vi "Run (G-Audio).vi"(8 "error in (no error)":errorcluster, 11 "Audio Output Queue":refnum<queue>) -> (0 "error out":errorcluster)   [LabVIEW 2020, in "Audio Output.lvlib"]
doc: "The main audio output loop.\n\n<b>Priority:</b> Time Critical\n<b>Execution System:</b> Instrument I/O"
uses:
  Audio Output.lvlib
  Audio Output Queue Type.ctl
  Audio Output Config.ctl
  Audio Output Info.ctl
  <vilib>/Dataflow_G/G-Audio/Controls/Audio Device Info.ctl
  <vilib>/Dataflow_G/G-Audio/Controls/Audio Device Type.ctl
  <vilib>/Dataflow_G/G-Audio/Controls/Audio Device Native Data Format.ctl
  <vilib>/Dataflow_G/G-Audio/Controls/Audio Device Format.ctl
  State.ctl
  <vilib>/Dataflow_G/G-Audio/Controls/Audio Device Config.ctl
  <vilib>/Dataflow_G/G-Audio/Controls/Audio Device Refnum.ctl
  Packed Libraries/Messaging.lvlibp/Message Cluster.ctl
  0d524fd1-6f2e-443a-bc5a-9f55547fbf75.vi
  df8da7fd-5bea-41c3-a497-f65be9ea8de3.vi
  3674f1a7-3d32-4f10-b3d2-182b6974db2a.vi
  <vilib>/Dataflow_G/G-Audio/Private/Result To Error.vi
  df8da7fd-5bea-41c3-a497-f65be9ea8de3.vi/4dfb5711-8d81-45a3-b3db-a84d40650863.vi
  df8da7fd-5bea-41c3-a497-f65be9ea8de3.vi/c8869513-30c6-44f2-a2d3-73232fe63870.vi
  <vilib>/Dataflow_G/G-Audio/Private/Audio Device Refnum To Value.vi
  3674f1a7-3d32-4f10-b3d2-182b6974db2a.vi/4dfb5711-8d81-45a3-b3db-a84d40650863.vi
  3674f1a7-3d32-4f10-b3d2-182b6974db2a.vi/c8869513-30c6-44f2-a2d3-73232fe63870.vi
  df8da7fd-5bea-41c3-a497-f65be9ea8de3.vi/4dfb5711-8d81-45a3-b3db-a84d40650863.vi/4b7b629c-2e91-4160-9820-a26af8f6e677.vi
  df8da7fd-5bea-41c3-a497-f65be9ea8de3.vi/c8869513-30c6-44f2-a2d3-73232fe63870.vi/4b7b629c-2e91-4160-9820-a26af8f6e677.vi
  3674f1a7-3d32-4f10-b3d2-182b6974db2a.vi/4dfb5711-8d81-45a3-b3db-a84d40650863.vi/4b7b629c-2e91-4160-9820-a26af8f6e677.vi
  3674f1a7-3d32-4f10-b3d2-182b6974db2a.vi/c8869513-30c6-44f2-a2d3-73232fe63870.vi/4b7b629c-2e91-4160-9820-a26af8f6e677.vi
  Packed Libraries/Globals.lvlibp/Constants.vi
  Packed Libraries/Globals.lvlibp/Debug.vi
  <vilib>/Utility/Data Type/Get Numeric Information.vi
  <vilib>/Utility/error.llb/Error Cluster From Error Code.vi
  Packed Libraries/Messaging.lvlibp
  Packed Libraries/Globals.lvlibp
  <vilib>/ptbypt/NI_PtbyPt.lvlib
  <vilib>/Dataflow_G/G-Audio/G-Audio.lvlib
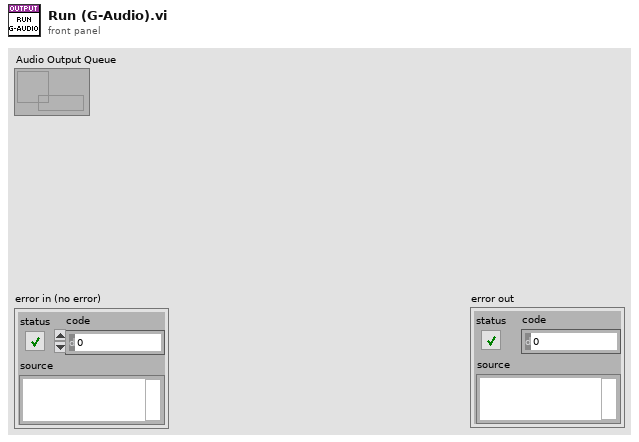
[diagram p1: front panel]
types:
  T1 = typedef "Audio Output.lvlib/Audio Output Config.ctl" = cluster{"Master":T2, "Headphones":T2}
  T2 = typedef "Audio Output.lvlib/Audio Output Info.ctl" = cluster{"Enable":bool, "Device Info":T3}
  T3 = typedef "G-Audio.lvlib/Audio Device Info.ctl" = cluster{"Name":string, "ID":u8[], "Device Type":T4, "Default":bool, "Native Data Formats":T5[]}
  T4 = typedef "G-Audio.lvlib/Audio Device Type.ctl" = enum16{"(None)", "Playback", "Capture", "Duplex", "Loopback"}
  T5 = typedef "G-Audio.lvlib/Audio Device Native Data Format.ctl" = cluster{"Format":T6, "Channels":u32, "Sample Rate (Hz)":u32, "Exclusive Mode":bool}
  T6 = typedef "G-Audio.lvlib/Audio Device Format.ctl" = enum16{"Native", "U8", "I16", "I32", "SGL"}
  T7 = typedef "Audio Output.lvlib/State.ctl" = enum16{"Init", "Configure", "Output", "Error", "Stop", "Idle", "Shutdown"}
  T8 = typedef "G-Audio.lvlib/Audio Device Config.ctl" = cluster{"Sample Rate (Hz)":u32, "Channels":u32, "Format":T6}
  T9 = typedef "G-Audio.lvlib/Audio Device Refnum.ctl" = refnum<file>
  T10 = typedef "Messaging.lvlibp/Message Cluster.ctl" = cluster{"Event":string, "Source":string, "Target":string, "Data":variant}
  T11 = typedef "Messaging.lvlib/Message Cluster.ctl" = cluster{"Event":string, "Source":string, "Target":string, "Data":variant}
  T12 = typedef "Audio Output.lvlib/Audio Output Queue Type.ctl" = cluster{"Master":waveform(i16)[], "Headphones":waveform(i16)[], "Start Time":dbl}
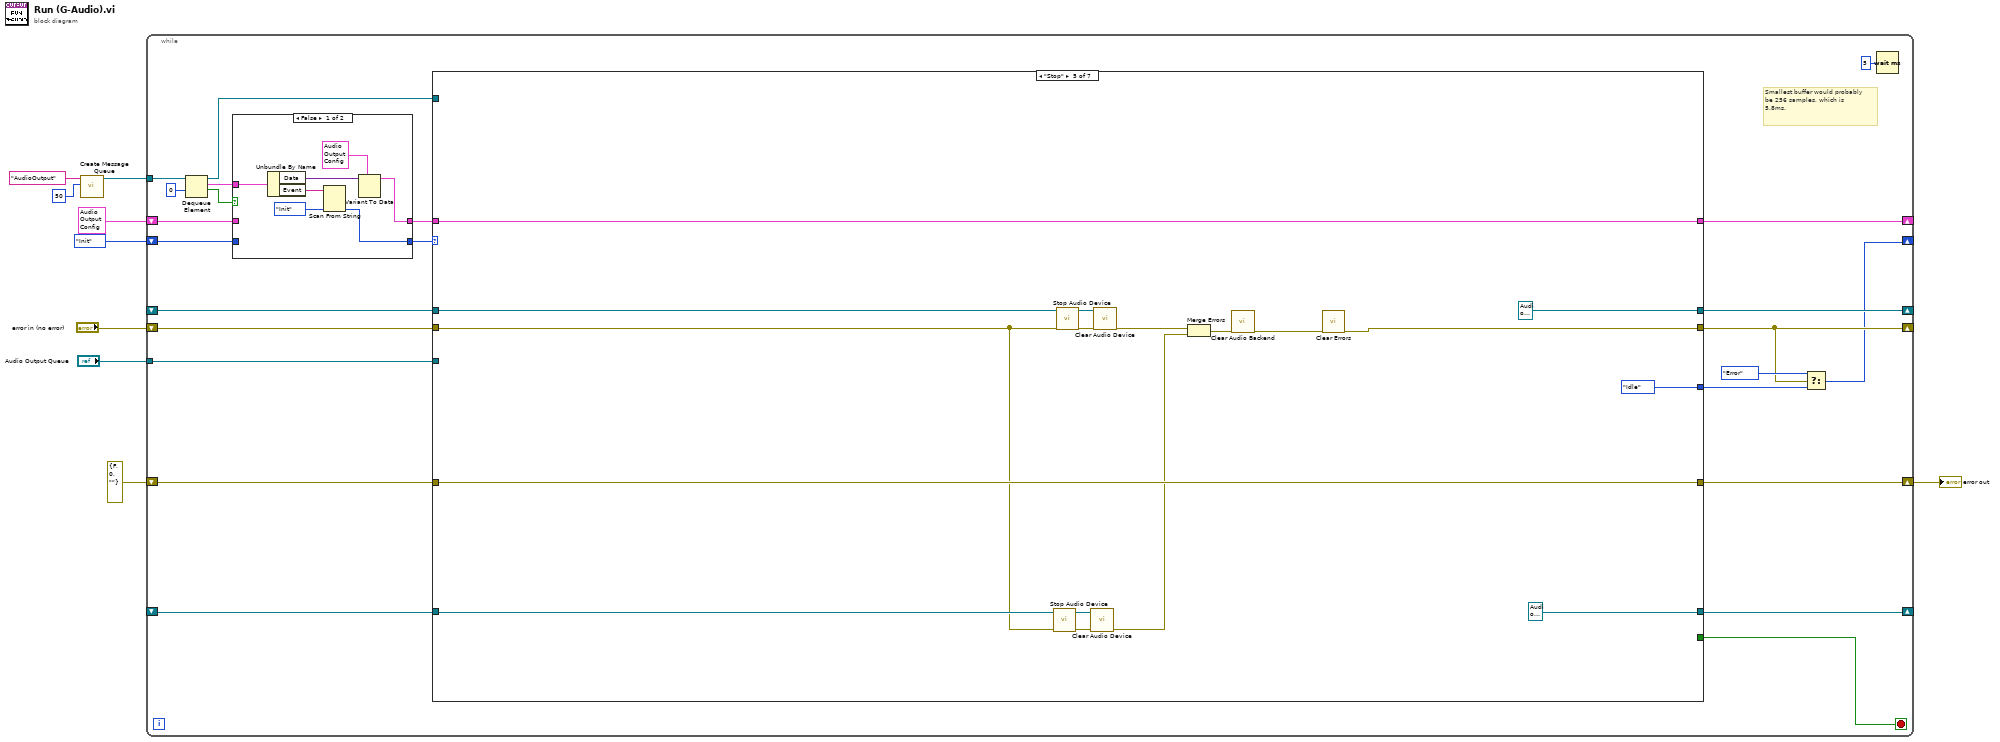
[diagram p0: block diagram]
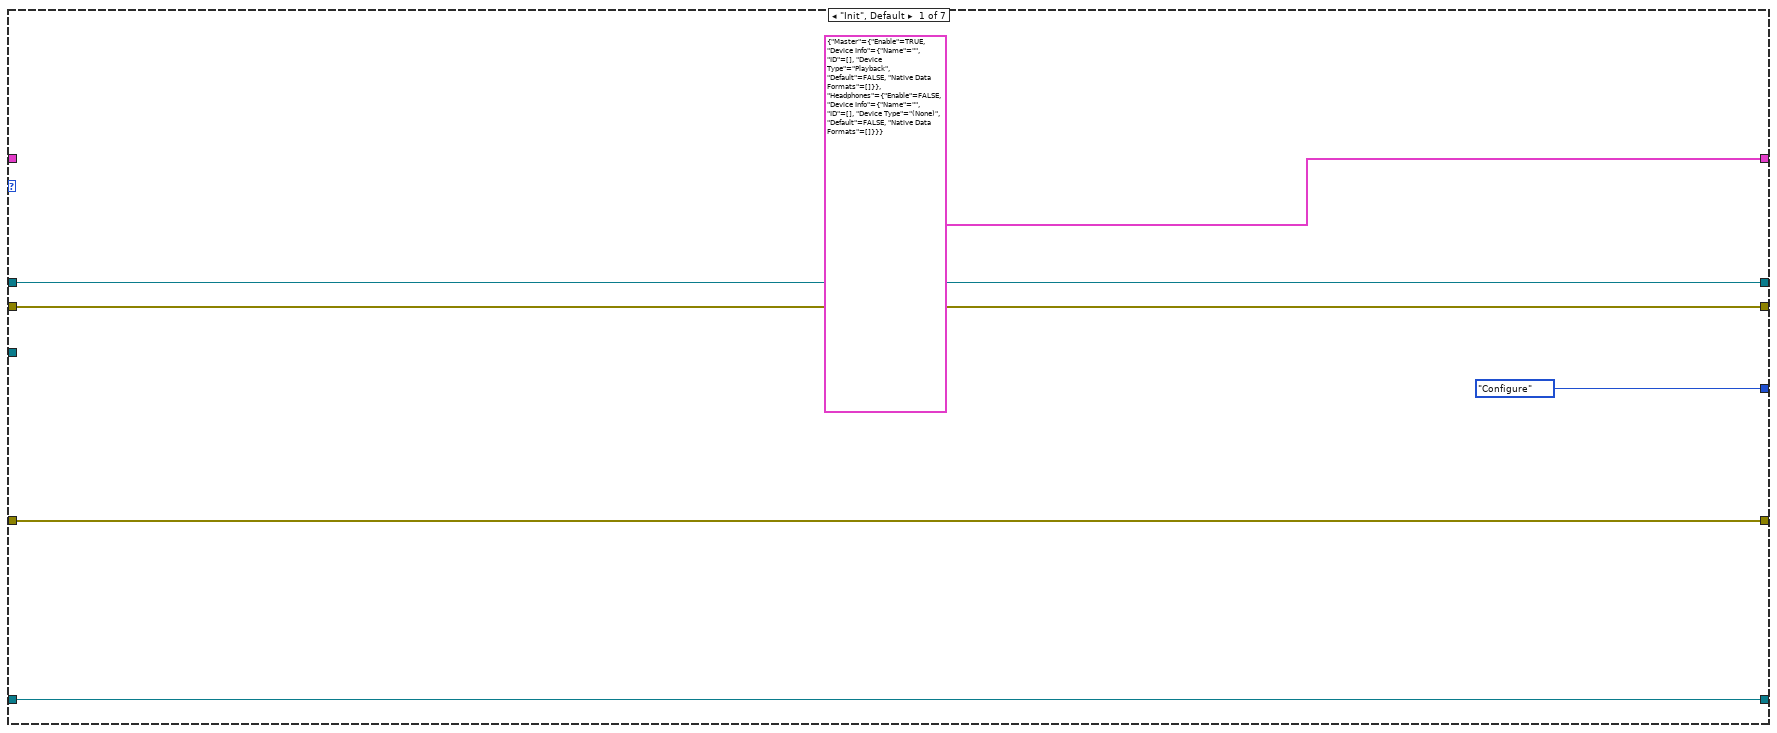
[diagram p3: hidden frame]
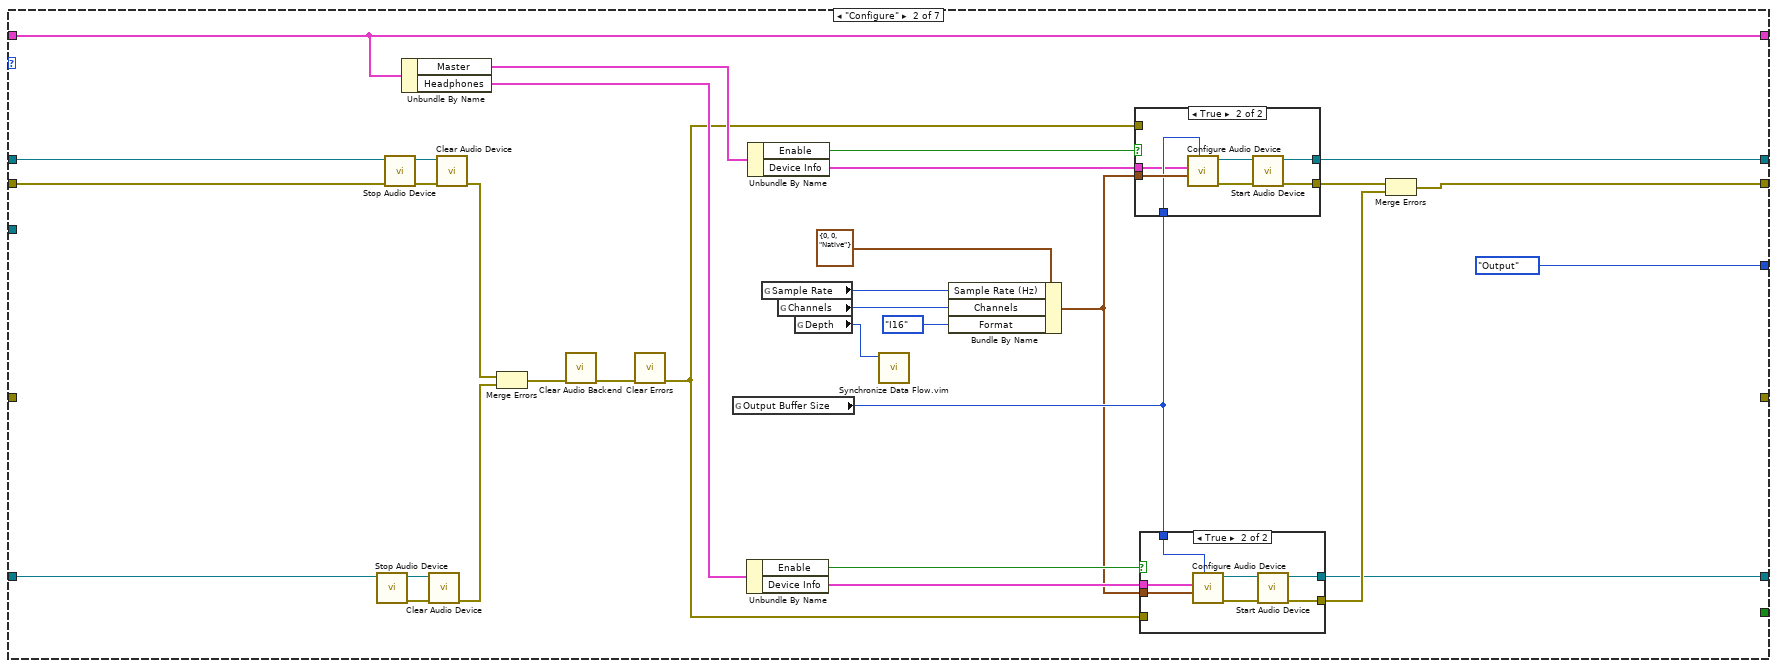
[diagram p4: hidden frame]
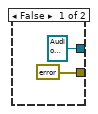
[diagram p5: hidden frame]
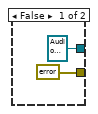
[diagram p6: hidden frame]
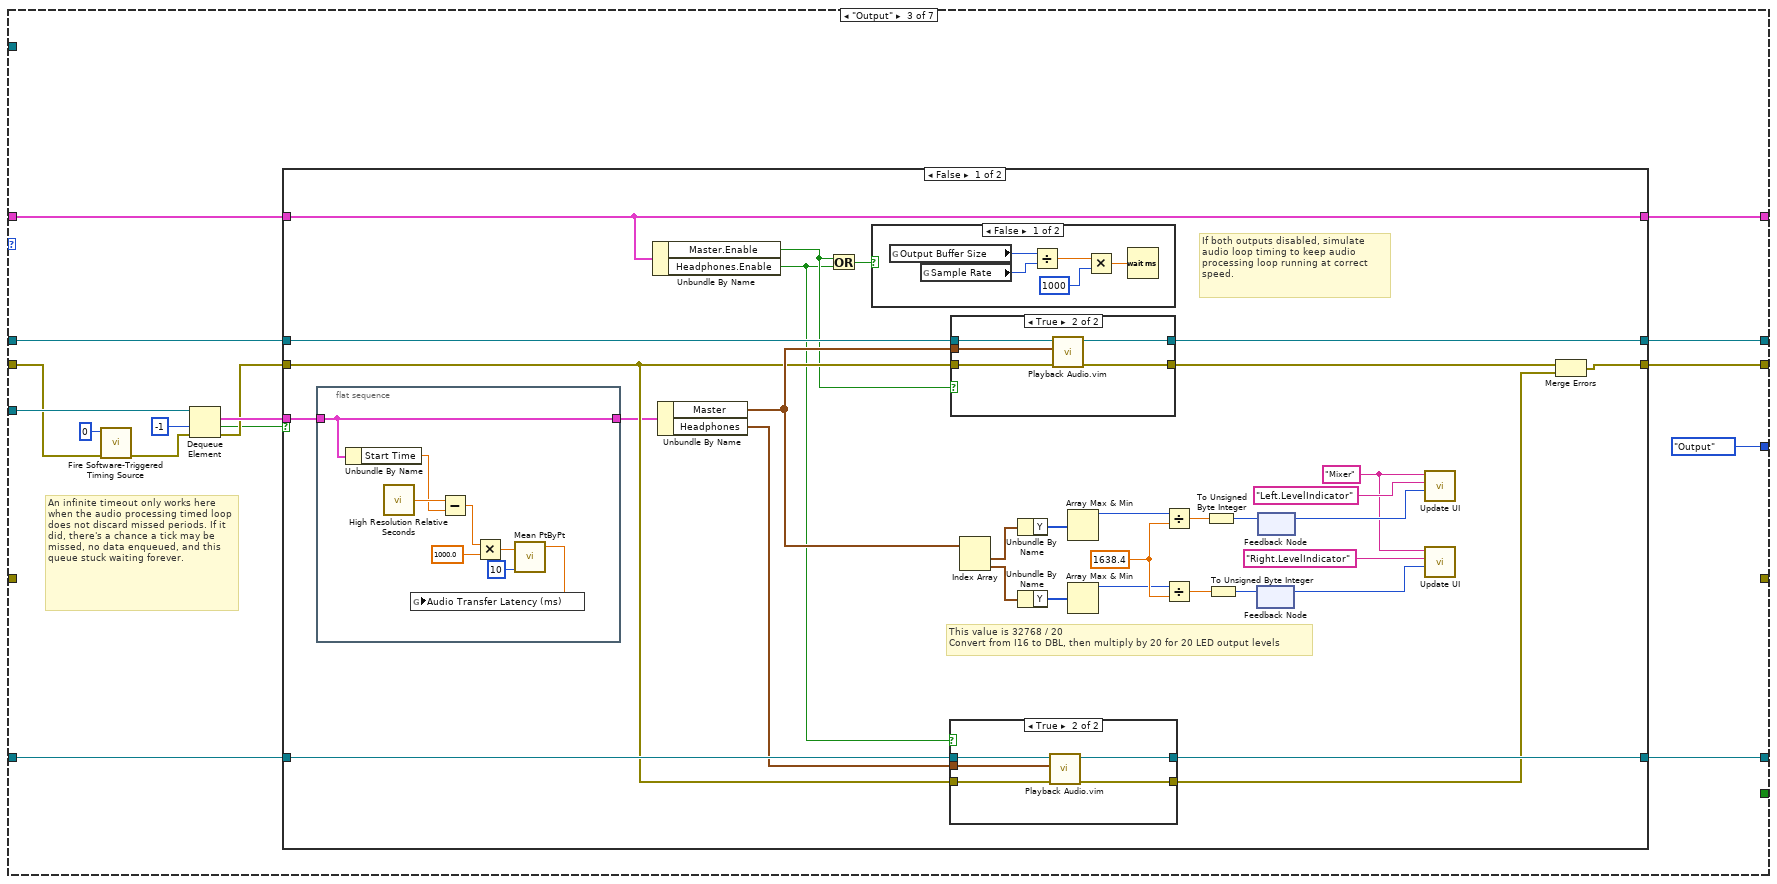
[diagram p7: hidden frame]
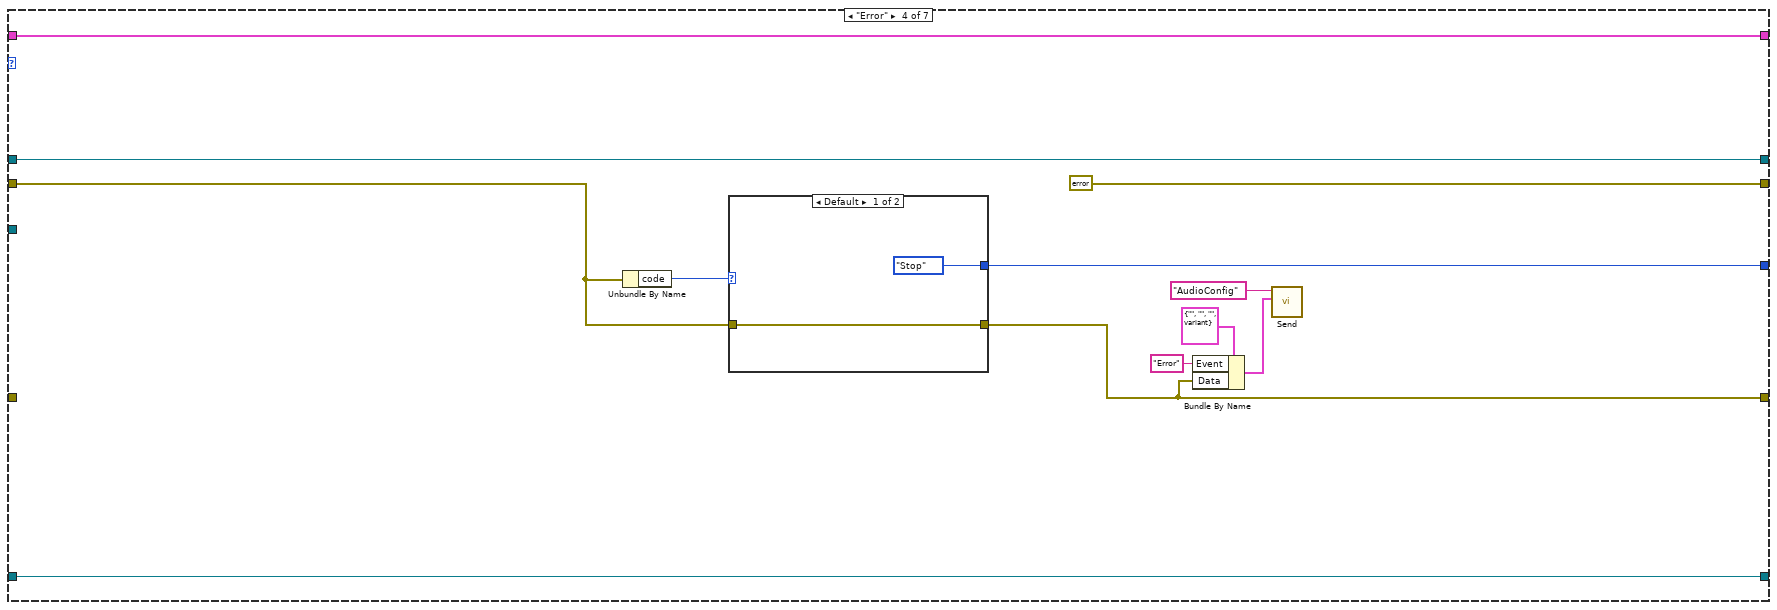
[diagram p12: hidden frame]
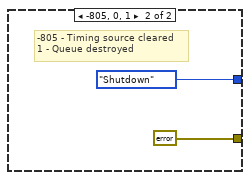
[diagram p13: hidden frame]
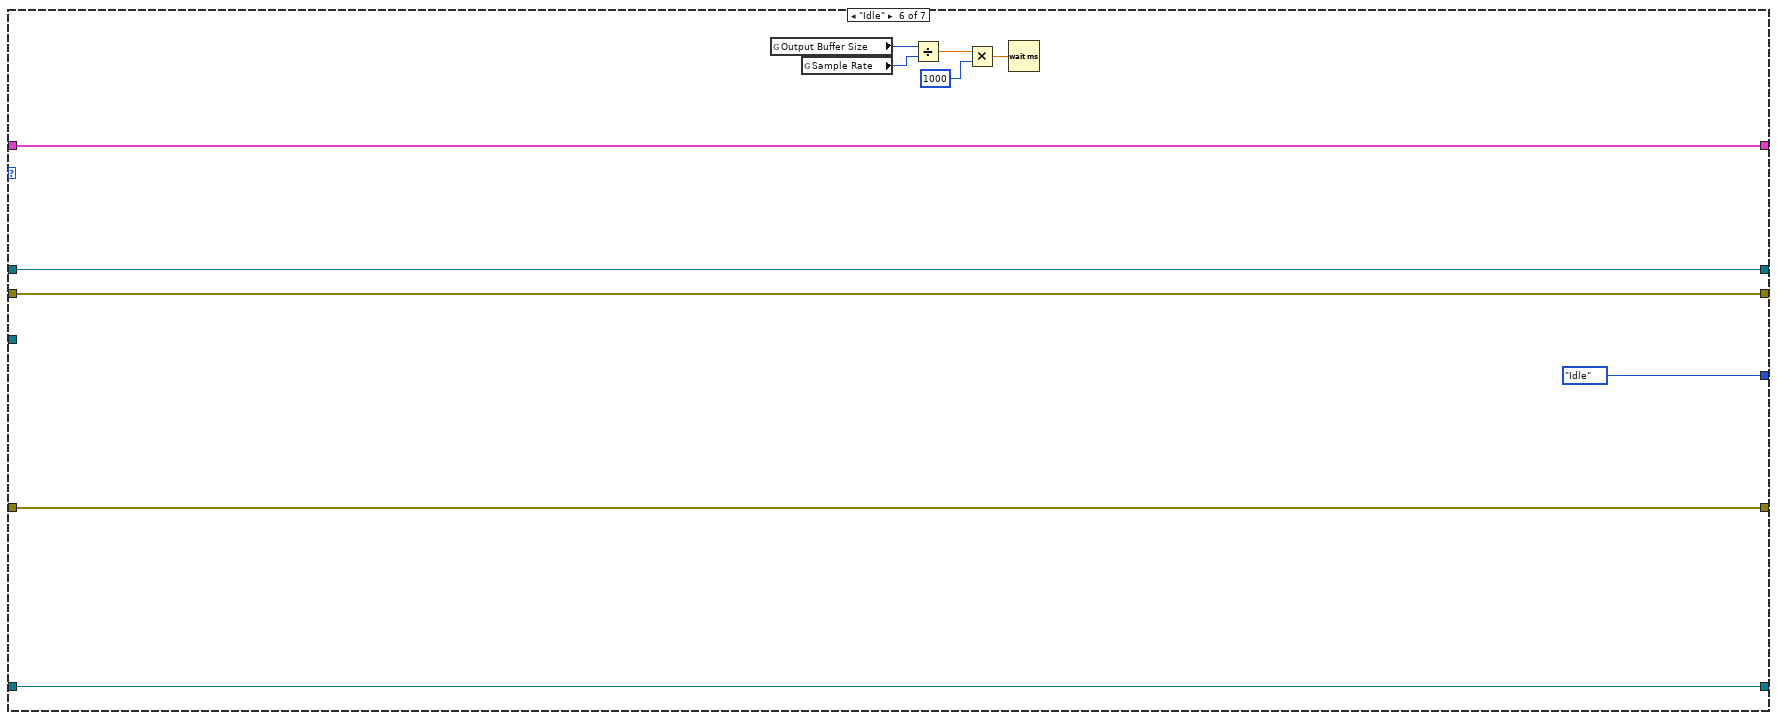
[diagram p14: hidden frame]
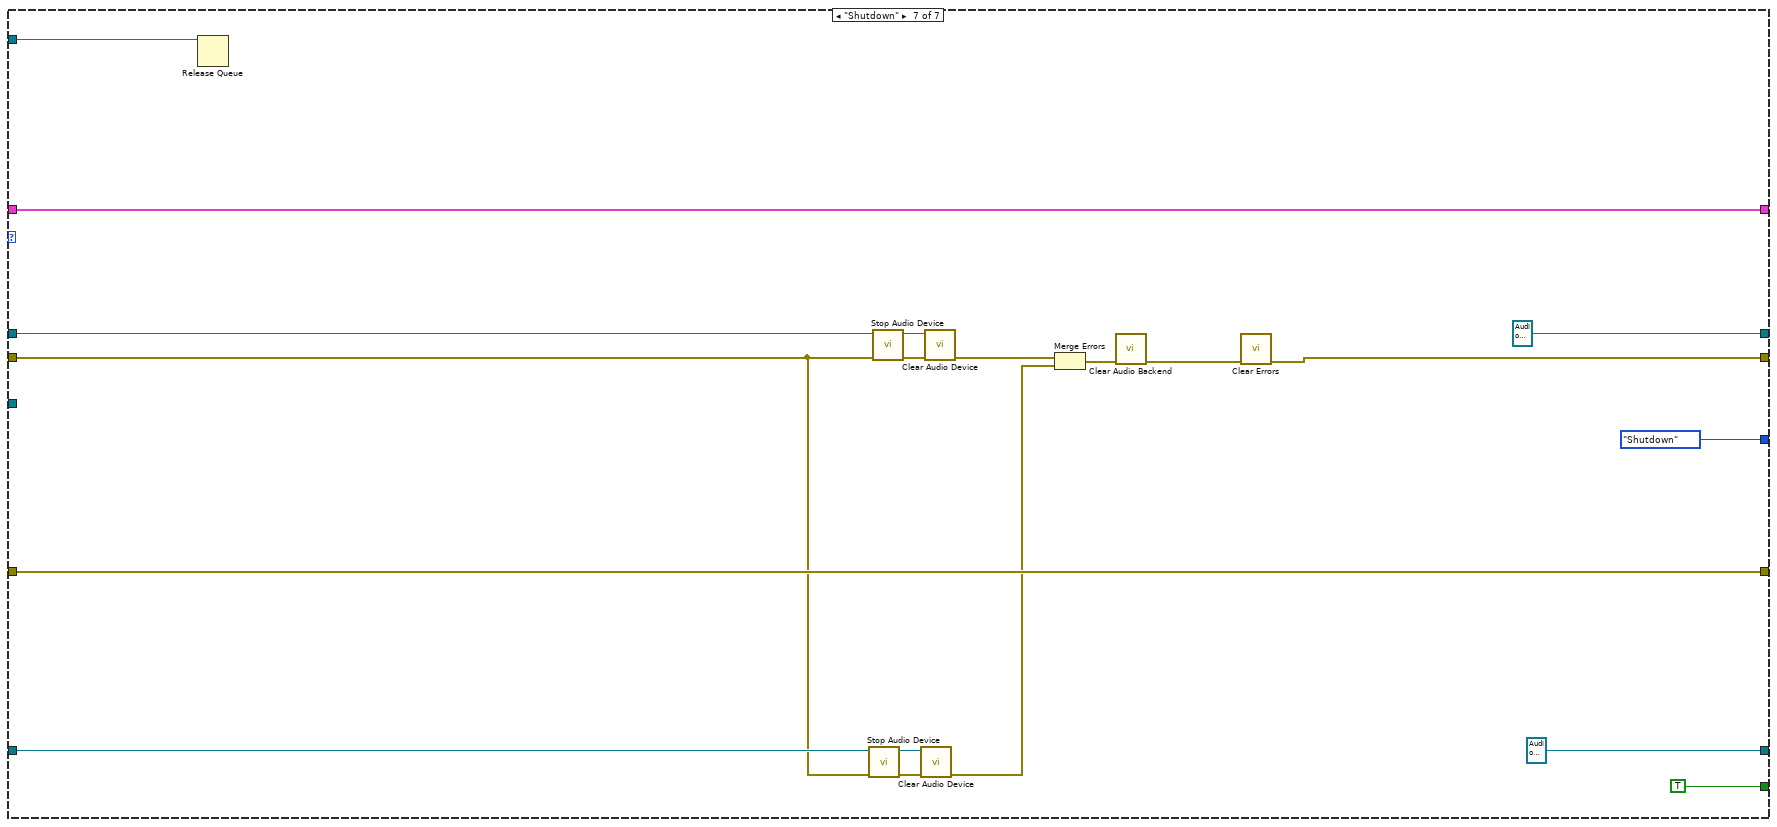
[diagram p15: hidden frame]
diagram:
  n1 = call "Create Message Queue.vi"("Max Size (1000)"=50, "Queue Name"="AudioOutput" ("name (unnamed)")) -> ("queue out"=w1:refnum<queue>)  [unwired: 8 in, 1 out]
  n2 = while {
    shift-right: [w28] -> _
    shift-left: State."Init" ("State") -> [w16]
    shift-right: [w33] -> _
    shift-left: _ -> [w32]
    shift-right: [w29] -> _
    shift-left: "error in (no error)" -> [w26]
    tunnel: "Audio Output Queue" -> [w24]
    shift-right: [w23] -> w7
    shift-left: errorcluster {"status"=FALSE, "code"=0, "source"=""} ("error out") -> [w22]
    shift-right: [w21] -> _
    shift-left: _ -> [w20]
    tunnel: w1 -> [w18]
    shift-right: [w10] -> _
    shift-left: T1 {"Master"={"Enable"=FALSE, "Device Info"={"Name"="", "ID"=[], "Device Type"=enum."(None)", "Default"=FALSE, "Native Data Formats"=[]}}, "Headphones"={"Enable"=FALSE, "Device Info"={"Name"="", "ID"=[], "Device Type"=enum."(None)", "Default"=FALSE, "Native Data Formats"=[]}}} -> [w12]
    stop <- w25 stop-if-true
    # "Smallest buffer would probably be 256 samples, which is 5.8ms."
    n3 = Dequeue Element(queue=w18, timeout in ms (-1)=0) -> (queue out=w13:refnum<queue>, element=w17:T11, timed out?=w14:bool)  [unwired: 1 in, 1 out]
    n4 = case shown="False" w14 {
      tunnel: w17 -> [w40 _]
      tunnel: w16 -> [_ w42]
      tunnel: [w37 w42] -> w15
      tunnel: [w34 w41] -> w11
      tunnel: w12 -> [_ w41]
      frame False {
        n5 = Unbundle By Name(w40) -> ("Data"=w35:variant, "Event"=w39:string)
        n6 = Scan From String(input string=w39, default 1=State."Init" ("State")) -> (output 1=w37:T7)  [unwired: 3 in, 3 out]
        n7 = Variant To Data(type=T1 {"Master"={"Enable"=FALSE, "Device Info"={"Name"="", "ID"=[], "Device Type"=enum."(None)", "Default"=FALSE, "Native Data Formats"=[]}}, "Headphones"={"Enable"=FALSE, "Device Info"={"Name"="", "ID"=[], "Device Type"=enum."(None)", "Default"=FALSE, "Native Data Formats"=[]}}}, Variant=w35) -> (data=w34:T1)  [unwired: 1 in, 1 out]
      }
      frame True {
      }
    }
    n8 = case shown="\"Stop\"" w15 {
      tunnel: [w47 w80 w112 w189 T9 refnum ("Audio Device Refnum Out") w219 T9 refnum ("Audio Device Refnum Out")] -> w33
      tunnel: w32 -> [w47 w66 w114 w189 w203 w219 w231]
      tunnel: [w46 w77 w113 errorcluster {"status"=FALSE, "code"=0, "source"=""} ("error out") w206 w218 w234] -> w29
      tunnel: [State."Configure" ("State") State."Output" ("State") State."Output" ("State") w183 State."Idle" ("State") State."Idle" ("State") State."Shutdown" ("State")] -> w31
      tunnel: w26 -> [w46 w63 w100 w186 w198 w218 w226]
      tunnel: [_ _ _ _ _ _ TRUE] -> w25
      tunnel: w24 -> [_ _ w108 _ _ _ _]
      tunnel: [w45 _ _ w179 w209 w217 w238] -> w23
      tunnel: w22 -> [w45 _ _ _ w209 w217 w238]
      tunnel: [w44 w57 w105 w185 T9 refnum ("Audio Device Refnum Out") w216 T9 refnum ("Audio Device Refnum Out")] -> w21
      tunnel: w20 -> [w44 w59 w104 w185 w199 w216 w227]
      tunnel: w13 -> [_ _ _ _ _ _ w237]
      tunnel: w11 -> [_ w73 w102 w184 w208 w221 w236]
      tunnel: [T1 {"Master"={"Enable"=TRUE, "Device Info"={"Name"="", "ID"=[], "Device Type"=enum."Playback", "Default"=FALSE, "Native Data Formats"=[]}}, "Headphones"={"Enable"=FALSE, "Device Info"={"Name"="", "ID"=[], "Device Type"=enum."(None)", "Default"=FALSE, "Native Data Formats"=[]}}} ("Audio Output Config") w73 w103 w184 w208 w221 w236] -> w10
      frame "Init", Default {
      }
      frame "Configure" {
        n9 = call <vilib>:"Stop Audio Device.vi"("Audio Device Refnum In"=w59) -> ("error out"=w61:errorcluster, "Audio Device Refnum Out"=w60:T9)  [unwired: 9 in]
        n10 = call <vilib>:"Stop Audio Device.vi"("error in (no error)"=w63, "Audio Device Refnum In"=w66) -> ("error out"=w64:errorcluster, "Audio Device Refnum Out"=w65:T9)  [unwired: 8 in]
        n11 = Unbundle By Name(w73) -> ("Master"=w76:T2, "Headphones"=w74:T2)
        n12 = call <vilib>:"Clear Audio Device.vi"("error in (no error)"=w61, "Audio Device Refnum In"=w60) -> ("error out"=w58:errorcluster)  [unwired: 9 in]
        n13 = call <vilib>:"Clear Audio Device.vi"("error in (no error)"=w64, "Audio Device Refnum In"=w65) -> ("error out"=w62:errorcluster)  [unwired: 9 in]
        n14 = Merge Errors(w62, w58) -> (w72:errorcluster)
        n15 = call <vilib>:"Clear Audio Backend.vi"("error in (no error)"=w72) -> ("error out"=w49:errorcluster)  [unwired: 10 in]
        n16 = call <vilib>:"Clear Errors.vi"("error in (no error)"=w49) -> ("error out"=w67:errorcluster)  [unwired: 5 in, 1 out]
        n17 = global read "Constants.vi" "Output Buffer Size"() -> (w53:i32)
        n18 = Unbundle By Name(w74) -> ("Enable"=w70:bool, "Device Info"=w69:T3)
        n19 = Unbundle By Name(w76) -> ("Enable"=w71:bool, "Device Info"=w75:T3)
        n20 = global read "Constants.vi" "Sample Rate"() -> (w55:i32)
        n21 = global read "Constants.vi" "Channels"() -> (w54:i32)
        n22 = global read "Constants.vi" "Depth"() -> (w50:i32)
        n23 = call "Synchronize Data Flow.vim"("input 1"=w50) -> ()  [unwired: 3 in, 4 out]
        n24 = Bundle By Name(cluster=T8 {"Sample Rate (Hz)"=0, "Channels"=0, "Format"=enum."Native"} ("Audio Device Config"), "Sample Rate (Hz)"=w55, "Channels"=w54, "Format"=Audio_Device_Format."I16") -> (w52:T8)
        n25 = case shown="True" w71 {
          tunnel: [T9 refnum ("Audio Device Refnum Out") w98] -> w80
          tunnel: [errorcluster {"status"=FALSE, "code"=0, "source"=""} ("error out") w94] -> w78
          tunnel: w75 -> [_ w92]
          tunnel: w67 -> [_ _]
          tunnel: w52 -> [_ w96]
          tunnel: w53 -> [_ w95]
          frame False {
          }
          frame True {
            n26 = call <vilib>:"Configure Audio Device.vi"("Buffer Size (4096)"=w95, "Device Config"=w96, "Audio Device"=w92) -> ("error out"=w93:errorcluster, "Audio Device Refnum"=w97:T9)  [unwired: 5 in, 2 out]
            n27 = call <vilib>:"Start Audio Device.vi"("error in (no error)"=w93, "Audio Device Refnum In"=w97) -> ("error out"=w94:errorcluster, "Audio Device Refnum Out"=w98:T9)  [unwired: 8 in]
          }
        }
        n28 = case shown="True" w70 {
          tunnel: [T9 refnum ("Audio Device Refnum Out") w89] -> w57
          tunnel: [errorcluster {"status"=FALSE, "code"=0, "source"=""} ("error out") w86] -> w68
          tunnel: w69 -> [_ w83]
          tunnel: w52 -> [_ w87]
          tunnel: w67 -> [_ _]
          tunnel: w53 -> [_ w85]
          frame False {
          }
          frame True {
            n29 = call <vilib>:"Configure Audio Device.vi"("Buffer Size (4096)"=w85, "Device Config"=w87, "Audio Device"=w83) -> ("error out"=w84:errorcluster, "Audio Device Refnum"=w88:T9)  [unwired: 5 in, 2 out]
            n30 = call <vilib>:"Start Audio Device.vi"("error in (no error)"=w84, "Audio Device Refnum In"=w88) -> ("error out"=w86:errorcluster, "Audio Device Refnum Out"=w89:T9)  [unwired: 8 in]
          }
        }
        n31 = Merge Errors(w78, w68) -> (w77:errorcluster)
      }
      frame "Output" {
        # "An infinite timeout only works here when the audio processing timed loop does not discard missed periods. If it did, there's a chance a tick may be missed, no data enqueued, and this queue stuck waiting forever."
        n32 = call <vilib>:"Fire Software-Triggered Timing Source.vi"("error in (no error)"=w100, "trigger ID"=u8 0) -> ("error out"=w101:errorcluster)  [unwired: 8 in, 1 out]
        n33 = Dequeue Element(queue=w108, timeout in ms (-1)=-1, error in (no error)=w101) -> (element=w110:T12, timed out?=w106:bool, error out=w107:errorcluster)  [unwired: 1 out]
        n34 = case shown="False" w106 {
          tunnel: w114 -> [w135 w177]
          tunnel: [w129 w176] -> w113
          tunnel: [w134 w177] -> w112
          tunnel: w110 -> [w116 _]
          tunnel: w107 -> [w125 w176]
          tunnel: [w133 w175] -> w105
          tunnel: w104 -> [w132 w175]
          tunnel: [w126 w174] -> w103
          tunnel: w102 -> [w126 w174]
          frame False {
            w119 = "Mixer" ("ID")
            w142 = 1638.4
            # "If both outputs disabled, simulate audio loop timing to keep audio processing loop running at correct speed."
            # "This value is 32768 / 20\nConvert from I16 to DBL, then multiply by 20 for 20 LED output levels"
            n35 = flat-sequence {
              tunnel: w116 -> [w154]
              tunnel: [w154] -> w115
              frame #0 {
                n36 = Unbundle By Name(w154) -> ("Start Time"=w152:dbl)
                n37 = call <vilib>:"High Resolution Relative Seconds.vi"() -> ("relative seconds"=w153:dbl)
                n38 = Subtract(x=w153, y=w152) -> (x-y=w151:dbl)
                n39 = Multiply(x=w151, y=1000.0) -> (x*y=w149:dbl)
                n40 = call <vilib>:"Mean PtByPt.vi"("x"=w149, "sample length"=10) -> ("mean"=w148:dbl)  [unwired: 2 in, 1 out]
                n41 = global write "Debug.vi" "Audio Transfer Latency (ms)"(w148) -> ()
              }
            }
            n42 = Unbundle By Name(w126) -> ("Master.Enable"=w124:bool, "Headphones.Enable"=w123:bool)
            n43 = Unbundle By Name(w115) -> ("Master"=w128:waveform(i16)[], "Headphones"=w127:waveform(i16)[])
            n44 = Or(x=w124, y=w123) -> (x .or. y?=w122:bool)
            n45 = case shown="False" w122 {
              frame False {
                n46 = global read "Constants.vi" "Output Buffer Size"() -> (w155:i32)
                n47 = global read "Constants.vi" "Sample Rate"() -> (w156:i32)
                n48 = Divide(x=w155, y=w156) -> (x/y=w158:dbl)
                n49 = Multiply(x=w158, y=1000) -> (x*y=w157:dbl)
                n50 = Wait (ms)(milliseconds to wait=w157) -> ()  [unwired: 1 out]
              }
              frame True {
              }
            }
            n51 = case shown="True" w123 {
              tunnel: [w161 w165] -> w133
              tunnel: w132 -> [w161 w162]
              tunnel: [w160 w163] -> w131
              tunnel: w127 -> [_ w166]
              tunnel: w125 -> [w160 w164]
              frame False {
              }
              frame True {
                n52 = call "Playback Audio.vim"("error in (no error)"=w164, "Audio Data"=w166, "Audio Device Refnum In"=w162) -> ("error out"=w163:errorcluster, "Audio Device Refnum Out"=w165:T9)  [unwired: 7 in]
              }
            }
            n53 = case shown="True" w124 {
              tunnel: w135 -> [w168 w169]
              tunnel: [w168 w173] -> w134
              tunnel: w125 -> [w167 w172]
              tunnel: [w167 w171] -> w130
              tunnel: w128 -> [_ w170]
              frame False {
              }
              frame True {
                n54 = call "Playback Audio.vim"("error in (no error)"=w172, "Audio Data"=w170, "Audio Device Refnum In"=w169) -> ("error out"=w171:errorcluster, "Audio Device Refnum Out"=w173:T9)  [unwired: 7 in]
              }
            }
            n55 = Index Array(array=w128) -> (element #1=w137:waveform(i16), element #2=w138:waveform(i16))  [unwired: 2 in]
            n56 = Unbundle By Name(w137) -> ("Y"=w136:i16[])
            n57 = Unbundle By Name(w138) -> ("Y"=w139:i16[])
            n58 = Array Max & Min(array=w136) -> (max value=w140:i16)  [unwired: 3 out]
            n59 = Array Max & Min(array=w139) -> (max value=w141:i16)  [unwired: 3 out]
            n60 = Divide(x=w140, y=w142) -> (x/y=w143:dbl)
            n61 = Divide(x=w141, y=w142) -> (x/y=w144:dbl)
            n62 = To Unsigned Byte Integer(number=w143) -> (unsigned 8bit integer=w145:u8)
            n63 = To Unsigned Byte Integer(number=w144) -> (unsigned 8bit integer=w146:u8)
            n64 = feedback #1() -> (w117:u8)  [unwired: 1 in]
            n65 = feedback-in #1(w146) -> ()
            n66 = feedback #2() -> (w120:u8)  [unwired: 1 in]
            n67 = feedback-in #2(w145) -> ()
            n68 = call "Update UI.vi"("Data"=w120, "Target"="Left.LevelIndicator", "ID"=w119) -> ()  [unwired: 8 in, 1 out]
            n69 = call "Update UI.vi"("Data"=w117, "Target"="Right.LevelIndicator", "ID"=w119) -> ()  [unwired: 8 in, 1 out]
            n70 = Merge Errors(w130, w131) -> (w129:errorcluster)
          }
          frame True {
          }
        }
      }
      frame "Error" {
        n71 = Unbundle By Name(w186) -> ("code"=w187:i32)
        n72 = case shown="Default" w187 {
          tunnel: w186 -> [w191 _]
          tunnel: [w191 errorcluster {"status"=FALSE, "code"=0, "source"=""} ("error out")] -> w179
          tunnel: [State."Stop" ("State") State."Shutdown" ("State")] -> w183
          frame Default {
          }
          frame -805, 0, 1 {
            # "-805 - Timing source cleared\n1 - Queue destroyed"
          }
        }
        n73 = Bundle By Name(cluster=T10 {"Event"="", "Source"="", "Target"="", "Data"=variant} ("Message"), "Event"="Error", "Data"=w179) -> (w180:T10)
        n74 = call "Send.vi"("Message"=w180, "Queue Name"="AudioConfig") -> ()  [unwired: 9 in, 1 out]
      }
      frame "Stop" {
        n75 = call <vilib>:"Stop Audio Device.vi"("error in (no error)"=w198, "Audio Device Refnum In"=w199) -> ("error out"=w201:errorcluster, "Audio Device Refnum Out"=w200:T9)  [unwired: 8 in]
        n76 = call <vilib>:"Stop Audio Device.vi"("error in (no error)"=w198, "Audio Device Refnum In"=w203) -> ("error out"=w204:errorcluster, "Audio Device Refnum Out"=w205:T9)  [unwired: 8 in]
        n77 = call <vilib>:"Clear Audio Device.vi"("error in (no error)"=w201, "Audio Device Refnum In"=w200) -> ("error out"=w197:errorcluster)  [unwired: 9 in]
        n78 = call <vilib>:"Clear Audio Device.vi"("error in (no error)"=w204, "Audio Device Refnum In"=w205) -> ("error out"=w202:errorcluster)  [unwired: 9 in]
        n79 = Merge Errors(w202, w197) -> (w207:errorcluster)
        n80 = call <vilib>:"Clear Audio Backend.vi"("error in (no error)"=w207) -> ("error out"=w196:errorcluster)  [unwired: 10 in]
        n81 = call <vilib>:"Clear Errors.vi"("error in (no error)"=w196) -> ("error out"=w206:errorcluster)  [unwired: 5 in, 1 out]
      }
      frame "Idle" {
        n82 = global read "Constants.vi" "Output Buffer Size"() -> (w211:i32)
        n83 = global read "Constants.vi" "Sample Rate"() -> (w212:i32)
        n84 = Divide(x=w211, y=w212) -> (x/y=w214:dbl)
        n85 = Multiply(x=w214, y=1000) -> (x*y=w213:dbl)
        n86 = Wait (ms)(milliseconds to wait=w213) -> ()  [unwired: 1 out]
      }
      frame "Shutdown" {
        n87 = Release Queue(queue=w237) -> ()  [unwired: 2 in, 3 out]
        n88 = call <vilib>:"Stop Audio Device.vi"("error in (no error)"=w226, "Audio Device Refnum In"=w227) -> ("error out"=w229:errorcluster, "Audio Device Refnum Out"=w228:T9)  [unwired: 8 in]
        n89 = call <vilib>:"Stop Audio Device.vi"("error in (no error)"=w226, "Audio Device Refnum In"=w231) -> ("error out"=w232:errorcluster, "Audio Device Refnum Out"=w233:T9)  [unwired: 8 in]
        n90 = call <vilib>:"Clear Audio Device.vi"("error in (no error)"=w229, "Audio Device Refnum In"=w228) -> ("error out"=w225:errorcluster)  [unwired: 9 in]
        n91 = call <vilib>:"Clear Audio Device.vi"("error in (no error)"=w232, "Audio Device Refnum In"=w233) -> ("error out"=w230:errorcluster)  [unwired: 9 in]
        n92 = Merge Errors(w230, w225) -> (w235:errorcluster)
        n93 = call <vilib>:"Clear Audio Backend.vi"("error in (no error)"=w235) -> ("error out"=w224:errorcluster)  [unwired: 10 in]
        n94 = call <vilib>:"Clear Errors.vi"("error in (no error)"=w224) -> ("error out"=w234:errorcluster)  [unwired: 5 in, 1 out]
      }
    }
    n95 = Select(t=State."Error" ("State"), s=w29, f=w31) -> (s? t:f=w28:T7)
    n96 = Wait (ms)(milliseconds to wait=u32 5 ("millisecond multiple")) -> ()  [unwired: 1 out]
  }
  "error out" <- w7
